vi "DSF.Engine.Transceiver Thread.Transfer Group.Parse.vi"(8 "error in (no error)":errorcluster, 10 "Transfer Group in":refnum<class "DSF.Engine.Transfer Group.lvclass">, 11 "Transceiver Thread in":refnum<class "DSF.Engine.Transceiver Thread.lvclass">) -> (0 "error out":errorcluster, 2 "Transfer Group out":refnum<class "DSF.Engine.Transfer Group.lvclass">, 3 "Transceiver Thread out":refnum<class "DSF.Engine.Transceiver Thread.lvclass">)   [LabVIEW 2017, in "Data Sharing Framework Engine.lvlib" / "DSF.Engine.Transceiver Thread.lvclass"]
uses:
  DSF.Engine.Transceiver Thread.lvclass
  Transfer/DSF.Engine.Transfer Group.lvclass
  Transfer/DSF.Engine.Transfer Group.lvclass/DSF.Engine.Transfer Group.ctl
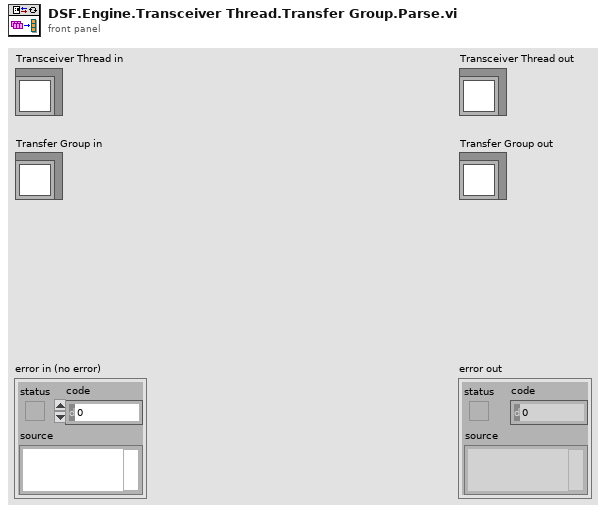
[diagram p1: front panel]
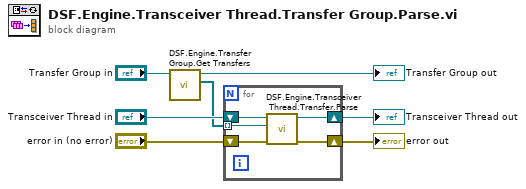
[diagram p0: block diagram]
diagram:
  n1 = call "DSF.Engine.Transfer Group.Get Transfers.vi"("Transfer Group in"="Transfer Group in") -> ("Transfers"=w5:refnum<class "DSF.Engine.Transfer.lvclass">[], "Transfer Group out"=→"Transfer Group out":refnum<class "DSF.Engine.Transfer Group.lvclass">)  [unwired: 9 in]
  n2 = for {
    tunnel: w5 -> [w8] mode=indexing
    shift-right: [w12] -> w4
    shift-left: "Transceiver Thread in" -> [w10]
    shift-right: [w11] -> w3
    shift-left: "error in (no error)" -> [w9]
    n3 = call "DSF.Engine.Transceiver Thread.Transfer.Parse.vi"("error in (no error)"=w9, "Transfer"=w8, "Transceiver Thread in"=w10) -> ("error out"=w11:errorcluster, "Transceiver Thread out"=w12:refnum<class "DSF.Engine.Transceiver Thread.lvclass">)  [unwired: 7 in]
  }
  "error out" <- w3
  "Transceiver Thread out" <- w4
